vi "Create Channel Task.vi"(8 "error in":errorcluster, 11 "NI Digital Input in":refnum<class "NI Digital Input.lvclass">) -> (0 "error out":errorcluster, 3 "NI Digital Input out":refnum<class "NI Digital Input.lvclass">)   [LabVIEW 2023, in "HardwareAbstractionLayer_LVOOP.lvlib" / "NI Digital Input.lvclass"]
doc: "This VI Analog Input Voltage Created the Task Physical Channel"
uses:
  NI Digital Input.lvclass
  NI Digital Input.lvclass/NI Digital Input.ctl
  <vilib>/DAQmx/create/channels.llb/DAQmx Create Channel (DI-Digital Input).vi
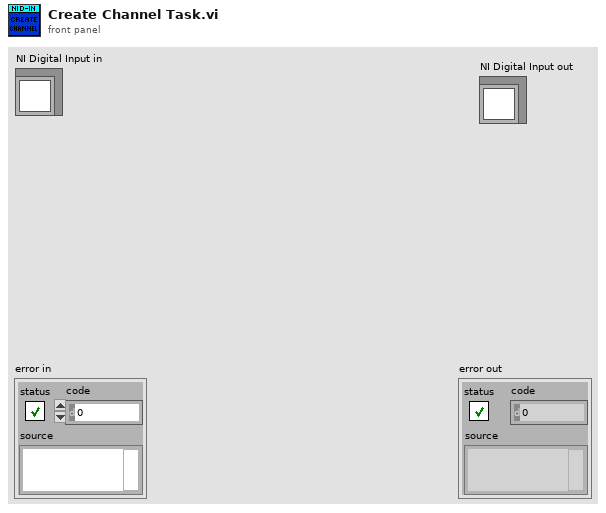
[diagram p1: front panel]
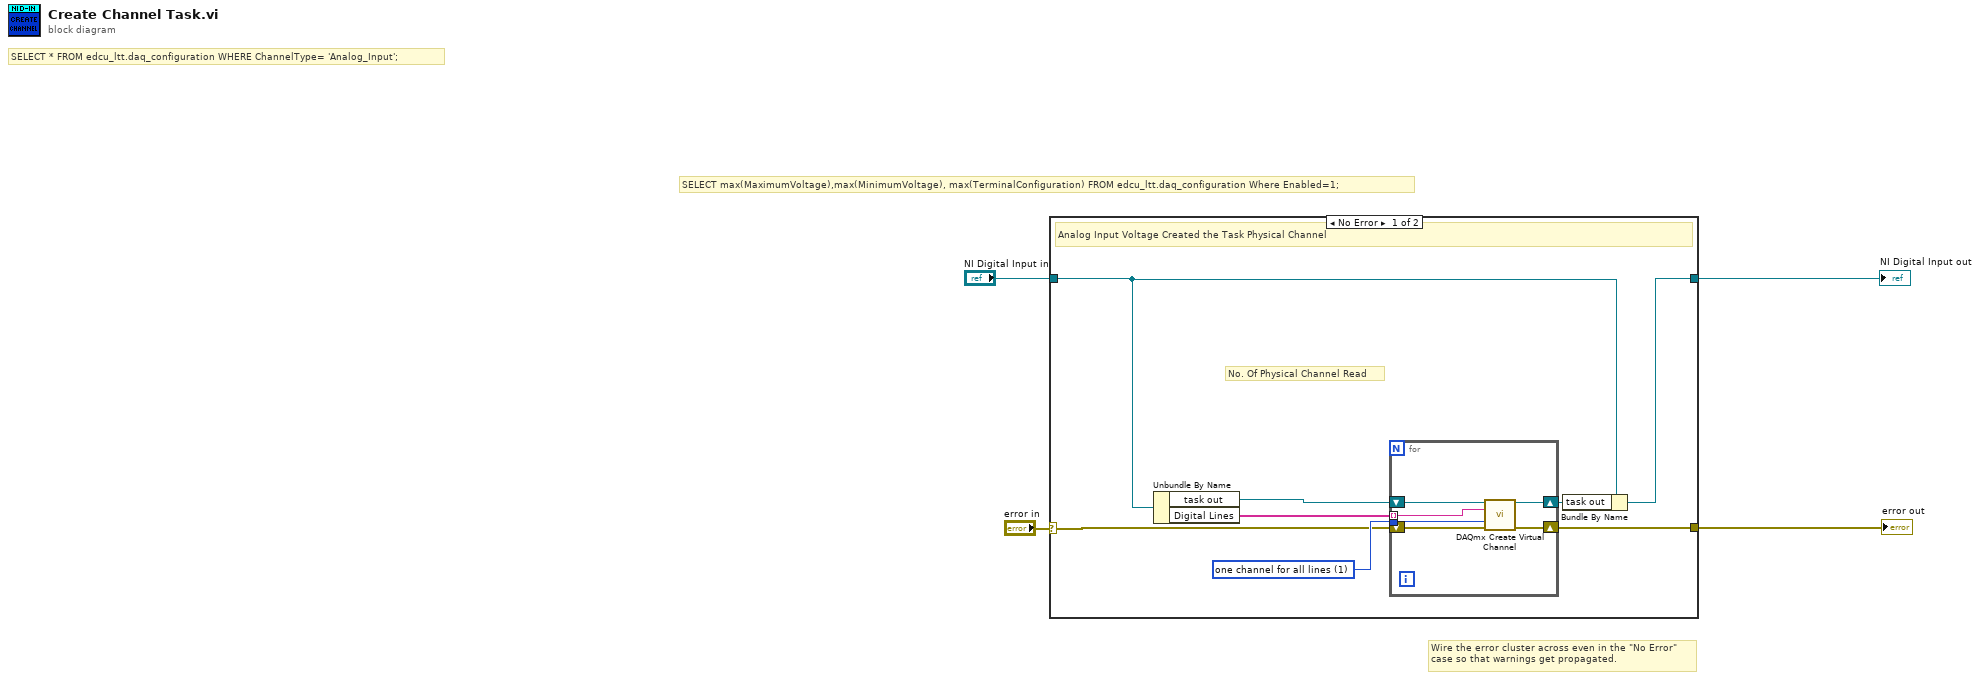
[diagram p0: block diagram]
diagram:
  # "SELECT max(MaximumVoltage),max(MinimumVoltage), max(TerminalConfiguration) FROM edcu_ltt.daq_configuration Where Enabled=1;"
  # "Wire the error cluster across even in the \"No Error\"\ncase so that warnings get propagated."
  # "SELECT * FROM edcu_ltt.daq_configuration WHERE ChannelType= 'Analog_Input';"
  n1 = case shown="No Error" "error in" {
    selector: "error in" -> [w6 w20]
    tunnel: [w8 w20] -> w3
    tunnel: [w11 w19] -> w1
    tunnel: "NI Digital Input in" -> [w12 w19]
    frame No Error {
      w9 = 1 items=["one channel for each line", "one channel for all lines"] ("line grouping")
      # "No. Of Physical Channel Read"
      # "Analog Input Voltage Created the Task Physical Channel"
      n2 = Unbundle By Name(w12) -> ("task out"=w10:refnum<k21>, "Digital Lines"=w5:tag[])
      n3 = for {
        tunnel: w9 -> [w17]
        shift-right: [w15] -> w7
        shift-left: w10 -> [w18]
        shift-right: [w16] -> w8
        shift-left: w6 -> [w14]
        tunnel: w5 -> [w13] mode=indexing
        n4 = call-poly <vilib>:"DAQmx Create Virtual Channel.vi"("task in"=w18, "lines"=w13, "line grouping"=w17, "error in"=w14) -> ("task out"=w15:refnum<k21>, "error out"=w16:errorcluster)  [unwired: 10 in]
      }
      n5 = Bundle By Name(cluster=w12, "task out"=w7) -> (w11:refnum<class "NI Digital Input.lvclass">)
    }
    frame Error {
    }
  }
  "error out" <- w3
  "NI Digital Input out" <- w1
